vi "ResetCountersHW.vi"(8 "error in (no error)":errorcluster, 11 "BME_DG_Base in":refnum<class "BME_DG_Base.lvclass">) -> (0 "error out":errorcluster, 3 "BME_DG_Base out":refnum<class "BME_DG_Base.lvclass">)   [LabVIEW 2009, in "POLARIS BME DG.lvlib" / "BME_DG_Base.lvclass"]
uses:
  BME_DG_Base.lvclass
  BME_DG_Base.lvclass/BME_DG_Base.ctl
  BME_DG_Chnl/BME_DG_Chnl.lvclass
  POLARIS BME DG.lvlib
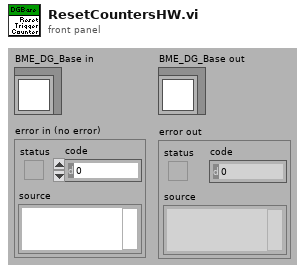
[diagram p1: front panel]
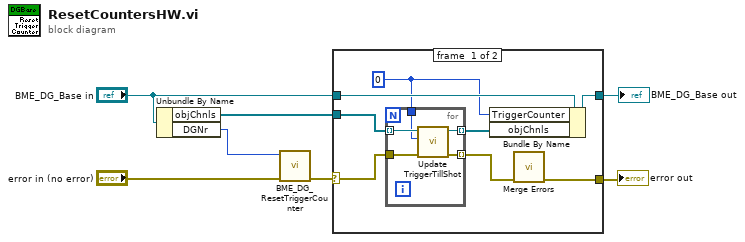
[diagram p0: block diagram]
diagram:
  n1 = Unbundle By Name("BME_DG_Base in") -> ("objChnls"=w3:refnum<class "BME_DG_Chnl.lvclass">[], "DGNr"=w1:i32)
  n2 = call "BME_DG_ResetTriggerCounter.vi"("error in (no error)"="error in (no error)", "DG_Number"=w1) -> ("error out"=w2:errorcluster)  [unwired: 8 in, 1 out]
  n3 = case shown="No Error" w2 {
    selector: w2 -> [w12 w21]
    tunnel: "BME_DG_Base in" -> [w15 w22]
    tunnel: [w14 w22] -> w5
    tunnel: [w8 w21] -> w4
    tunnel: w3 -> [w13 _]
    frame #0 {
      w11 = 0 ("TriggerCounter")
      n4 = for {
        tunnel: w13 -> [w20] mode=indexing
        tunnel: w12 -> [w19]
        tunnel: w11 -> [w18]
        tunnel: [w17] -> w10 mode=indexing
        tunnel: [w16] -> w9 mode=indexing
        n5 = call-dynamic "Update TriggerTillShot.vi"("error in (no error)"=w19, "TriggerCounter"=w18, "BME_DG_Chnl in"=w20) -> ("error out"=w16:errorcluster, "BME_DG_Chnl out"=w17:refnum<class "BME_DG_Chnl.lvclass">)  [unwired: 5 in, 2 out]
      }
      n6 = Bundle By Name(cluster=w15, "TriggerCounter"=w11, "objChnls"=w10) -> (w14:refnum<class "BME_DG_Base.lvclass">)
      n7 = call <vilib>:"Merge Errors.vi"("error array in"=w9) -> ("error out"=w8:errorcluster)  [unwired: 6 in]
    }
    frame #1 {
    }
  }
  "error out" <- w4
  "BME_DG_Base out" <- w5
